vi "SimpleWinFormControl.vi"() -> ()   [LabVIEW 2020]
uses:
  D:/dev/WinFormsApp/WinFormsControls/bin/Release/WinFormsControls.dll
panel:
  out "Text":string
  out "Is Checked?":bool
  out "error out":errorcluster
  in  "stop":bool
  in  "MyControl":refnum<k24>(container)
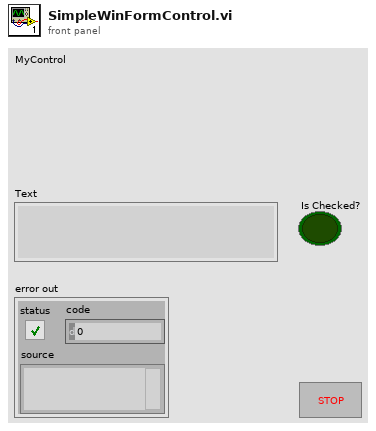
[diagram p1: front panel]
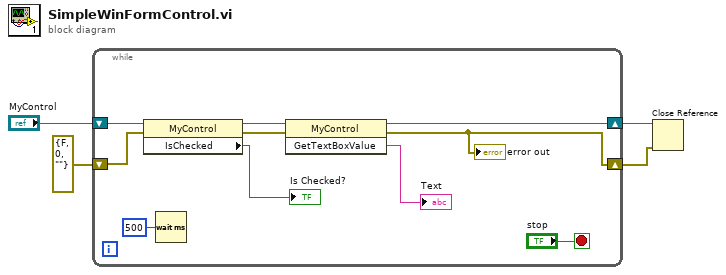
[diagram p0: block diagram]
diagram:
  n1 = while {
    shift-right: [w11] -> w1
    shift-left: "MyControl" -> [w13]
    shift-right: [w8] -> w2
    shift-left: errorcluster {"status"=FALSE, "code"=0, "source"=""} ("error out") -> [w10]
    stop <- "stop" stop-if-true
    n2 = property class="MyControl"(reference=w13) -> (reference out=w7:refnum<k24>, "IsChecked"=→"Is Checked?":bool)  [unwired: 1 in, 1 out]
    n3 = Wait (ms)(milliseconds to wait=u32 500) -> ()  [unwired: 1 out]
    n4 = invoke class="MyControl" method="GetTextBoxValue"(reference=w7, error in=w10) -> (reference out=w11:refnum<k24>, error out=w8:errorcluster, "GetTextBoxValue"=→"Text":string)  [unwired: 1 in]
    "error out" <- w8
  }
  n5 = Close Reference(reference=w1, error in (no error)=w2) -> ()  [unwired: 1 out]
